vi "Get TCP Settings.vi"(8 "error in (no error)":errorcluster, 11 "Item Ref in":T1 format="%.0x") -> (0 "error out":errorcluster, 1 "Port":u16, 2 "Address":string, 3 "Item Ref out":T1 format="%.0x", 5 "Timeout":i32)   [LabVIEW 2020, in "Modbus Master System Explorer.lvlib"]
uses:
  Modbus Master System Explorer.lvlib
  <vilib>/NI VeriStand/Custom Device API/Custom Device Item Ref.ctl
  Shared/Constants.vi
  <vilib>/NI VeriStand/Custom Device API/Get Item Property (String).vi
  <vilib>/NI VeriStand/Custom Device API/Get Item Property (U16).vi
  <vilib>/NI VeriStand/Custom Device API/Get Item Property (I32).vi
  Shared/Modbus Master Shared.lvlib
  <vilib>/NI VeriStand/Custom Device API/Custom Device API.lvlib
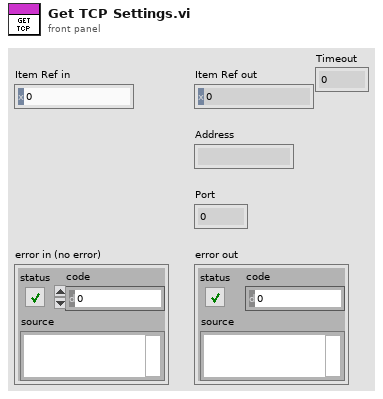
[diagram p1: front panel]
types:
  T1 = typedef "Custom Device API.lvlib/Custom Device Item Ref.ctl" = u64
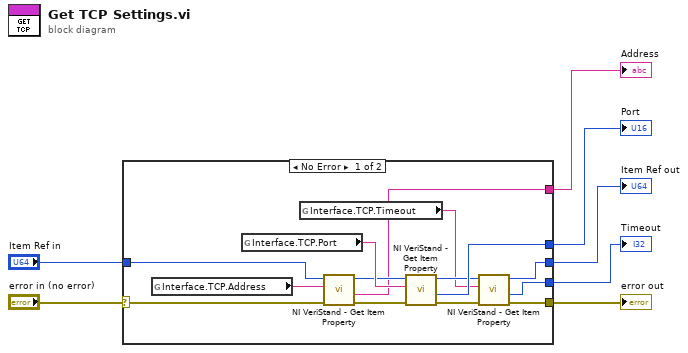
[diagram p0: block diagram]
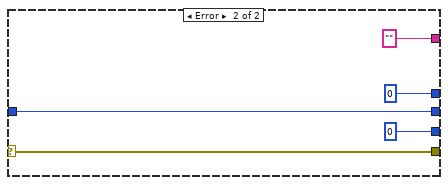
[diagram p2: hidden frame]
diagram:
  n1 = case shown="No Error" "error in (no error)" {
    selector: "error in (no error)" -> [w16 w25]
    tunnel: [w8 w25] -> w7
    tunnel: [w12 w26] -> w6
    tunnel: "Item Ref in" -> [w17 w26]
    tunnel: [w15 "" ("Value")] -> w3
    tunnel: [w14 u16 0 ("Value")] -> w2
    tunnel: [w10 0 ("Value")] -> w1
    frame No Error {
      n2 = global read "Constants.vi" "Interface.TCP.Address"() -> (w18:string)
      n3 = global read "Constants.vi" "Interface.TCP.Port"() -> (w21:string)
      n4 = global read "Constants.vi" "Interface.TCP.Timeout"() -> (w11:string)
      n5 = call-poly <vilib>:"NI VeriStand - Get Item Property.vi"("error in (no error)"=w16, "Property Name"=w18, "Item Ref in"=w17) -> ("error out"=w19:errorcluster, "Value"=w15:string, "Item Ref out"=w20:T1)  [unwired: 5 in, 1 out]
      n6 = call-poly <vilib>:"NI VeriStand - Get Item Property.vi"("error in (no error)"=w19, "Property Name"=w21, "Item Ref in"=w20) -> ("error out"=w9:errorcluster, "Value"=w14:u16, "Item Ref out"=w13:T1)  [unwired: 5 in, 1 out]
      n7 = call-poly <vilib>:"NI VeriStand - Get Item Property.vi"("error in (no error)"=w9, "Property Name"=w11, "Item Ref in"=w13) -> ("error out"=w8:errorcluster, "Value"=w10:i32, "Item Ref out"=w12:T1)  [unwired: 5 in, 1 out]
    }
    frame Error {
    }
  }
  "error out" <- w7
  "Item Ref out" <- w6
  "Port" <- w2
  "Address" <- w3
  "Timeout" <- w1
